vi "4Pi Focus Lock.vi"() -> ()   [LabVIEW 2016]
uses:
  4Pi Focus Lock Controls/4Pi Focus Lock - Notifier Type.ctl
  4Pi Focus Lock Controls/4Pi Focus Lock - Actions.ctl
  <vilib>/vision/Image Controls.llb/IMAQ Image.ctl
  Hardware Configuration/Hardware Configuration Controls/Device Type.ctl
  Hardware Configuration/Hardware Configuration Controls/Device Function.ctl
  Device Library/Cameras/Camera Controls/Generic Camera ROI.ctl
  Device Library/Cameras/Camera Controls/Generic Camera Actions.ctl
  Device Library/Stages/Stages Controls/Stage Actions.ctl
  <vilib>/addons/control/pid/pid.llb/PID (DBL).vi
  <vilib>/vision/NI_Vision_Development_Module.lvlib
  <vilib>/addons/control/pid/NI_PID_pid.lvlib
panel:
  in  "Z Drift Threshold (µm)":dbl=2.0
  in  "Z Move Limit (µm)":dbl=2.0
  out "Z Move":bool
  in  "Update Scale Factor":dbl=2.0
  out "dz (µm)":dbl format="%.2f"
  out "dt (s)":dbl format="%.3f"
  out "Measured Z (µm)":dbl=1.0 format="%.3g"
  out "Target Z (µm)":dbl=1.0 format="%.3g"
  out "Stage Position (µm)":dbl=1.0 format="%.2g"
  in  "Quit":bool
  in  "Sample Z Step No.":u32=2
  in  "Sample Z Step Size (µm)":dbl=2.0
  in  "D (Derivative)":dbl
  in  "I (Integral)":dbl
  in  "P (Proportional)":dbl=2.0
  in  "Set Camera ROI":bool
  out "Z Target and Fit Value (µm)":T1(graph)
  in  "Start Lock":bool
  # "PID Control Values"
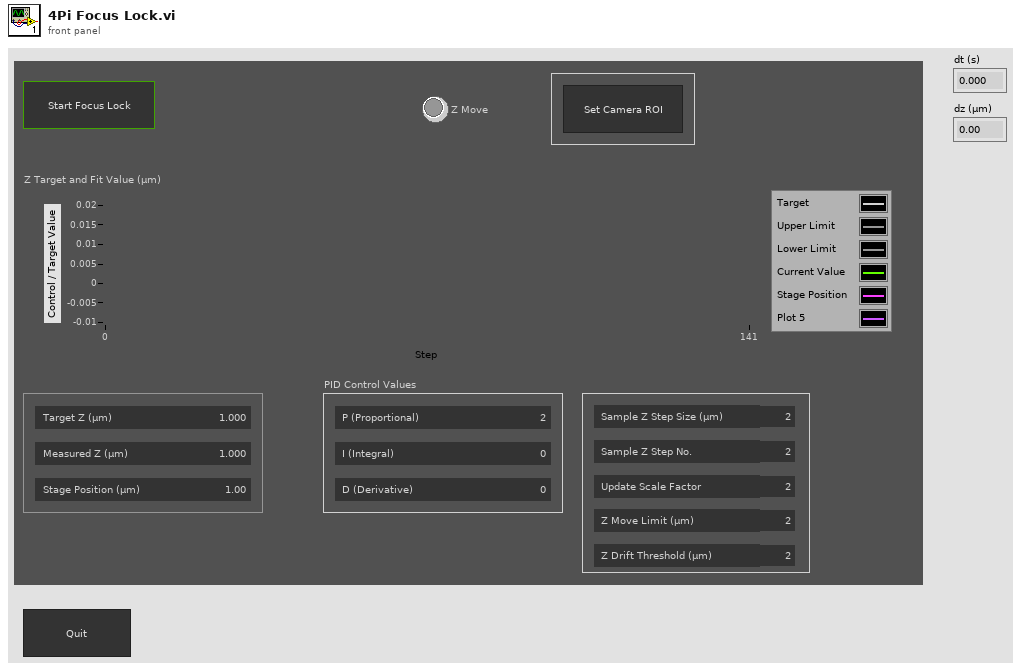
[diagram p1: front panel]
types:
  T1 = cluster{"Target 01":dbl, dbl, dbl, "Current 01":dbl, "Stage Position":dbl}
  T2 = typedef "4Pi Focus Lock - Actions.ctl" = enum16{"Idle", "Start Lock", "Restart Lock", "Get Target Position", "Get Ref Stack", "Cal Ref FFT", "Move To Init Z", "Start Primary Camera", "Get Current Position", "Get Current Position 1", "Get Actual Position", "Check Drift", "Move Z", "Update Plots", "Delay", "Abort", "Exit Loop", "Quit"}
  T3 = typedef "4Pi Focus Lock - Notifier Type.ctl" = cluster{"Actions":T2, "Z Drift Threshold":dbl, "Z Stage Move Limit (µm)":dbl, "Abort If Error":bool, "Z Correction Active":bool, "PID Values":dbl[], "Running?":bool, "Update Delay (ms)":i32, "Z Step Size (µm)":dbl, "Z Step No.":u32, "No. of Frames":u32, "Ref Stack (SGL)":T4[], "Cur Image (SGL)":T4, "Tmp Image FFT (CSG) ":T4, "Cur Image FFT (CSG) ":T4, "CC Image (SGL) ":T4, "Sample Z (µm)":dbl[], "Initial Z Position (µm)":dbl, "Ref FFT Stack (CSG)":T4[], "Tmp Image1 FFT (CSG) ":T4}
  T4 = typedef "IMAQ Image.ctl" = refnum<image>
  T5 = typedef "Image Type" = u32
  T6 = typedef "Device Function.ctl" = enum16{"Primary", "Secondary", "Overview", "Wide Field Drift Correction", "642 nm Excitation", "560 nm Excitation", "940 nm Excitation", "546 nm Excitation", "488 nm Excitation", "405 nm Excitation", "Objective Drift Correction", "4Pi Focus Lock", "4Pi Objective Lock", "Objective XY", "Objective Z", "Sample XY", "Sample Coarse Z", "Sample Z", "4Pi Lower", "4Pi Upper", "Mojo", "Adj Cavity", "Line Scanning", "Alert"}
  T7 = typedef "Device Type.ctl" = enum16{"AOTF", "Camera", "Deformable Mirror", "Laser", "Shutter", "Stage", "Waveform", "FPGA", "Email"}
  T8 = typedef "Stage Actions.ctl" = enum16{"Get Position", "MVR", "MOVE", "HALT", "ONTARGET", "ERROR", "REFERENCE", "INIT", "VELOCITY", "STATUS", "EXIT", "HOME", "ZEROPOS", "NANOPOS", "ANALOG", "QUIT"}
  T9 = typedef "Generic Camera Actions.ctl" = enum16{"Status", "Live Preview", "Capture", "Abort", "Set Exposure Time (s)", "Get Exposure Time (s)", "Record Settings", "Set ROI", "Get ROI", "Defect Correction On/Off", "Cooler On/Off", "Fan On/Off", "Quit"}
  T10 = typedef "Generic Camera ROI.ctl" = cluster{"H_Offset":u16, "V_Offset":u16, "H_Width":u16, "V_Width":u16}
  T11 = typedef "Stage Status.ctl" = enum16{"Error", "Abort", "Busy", "On Target"}
  T12 = cluster{"PID Values[0]":dbl, "PID Values[1]":dbl, "PID Values[2]":dbl}
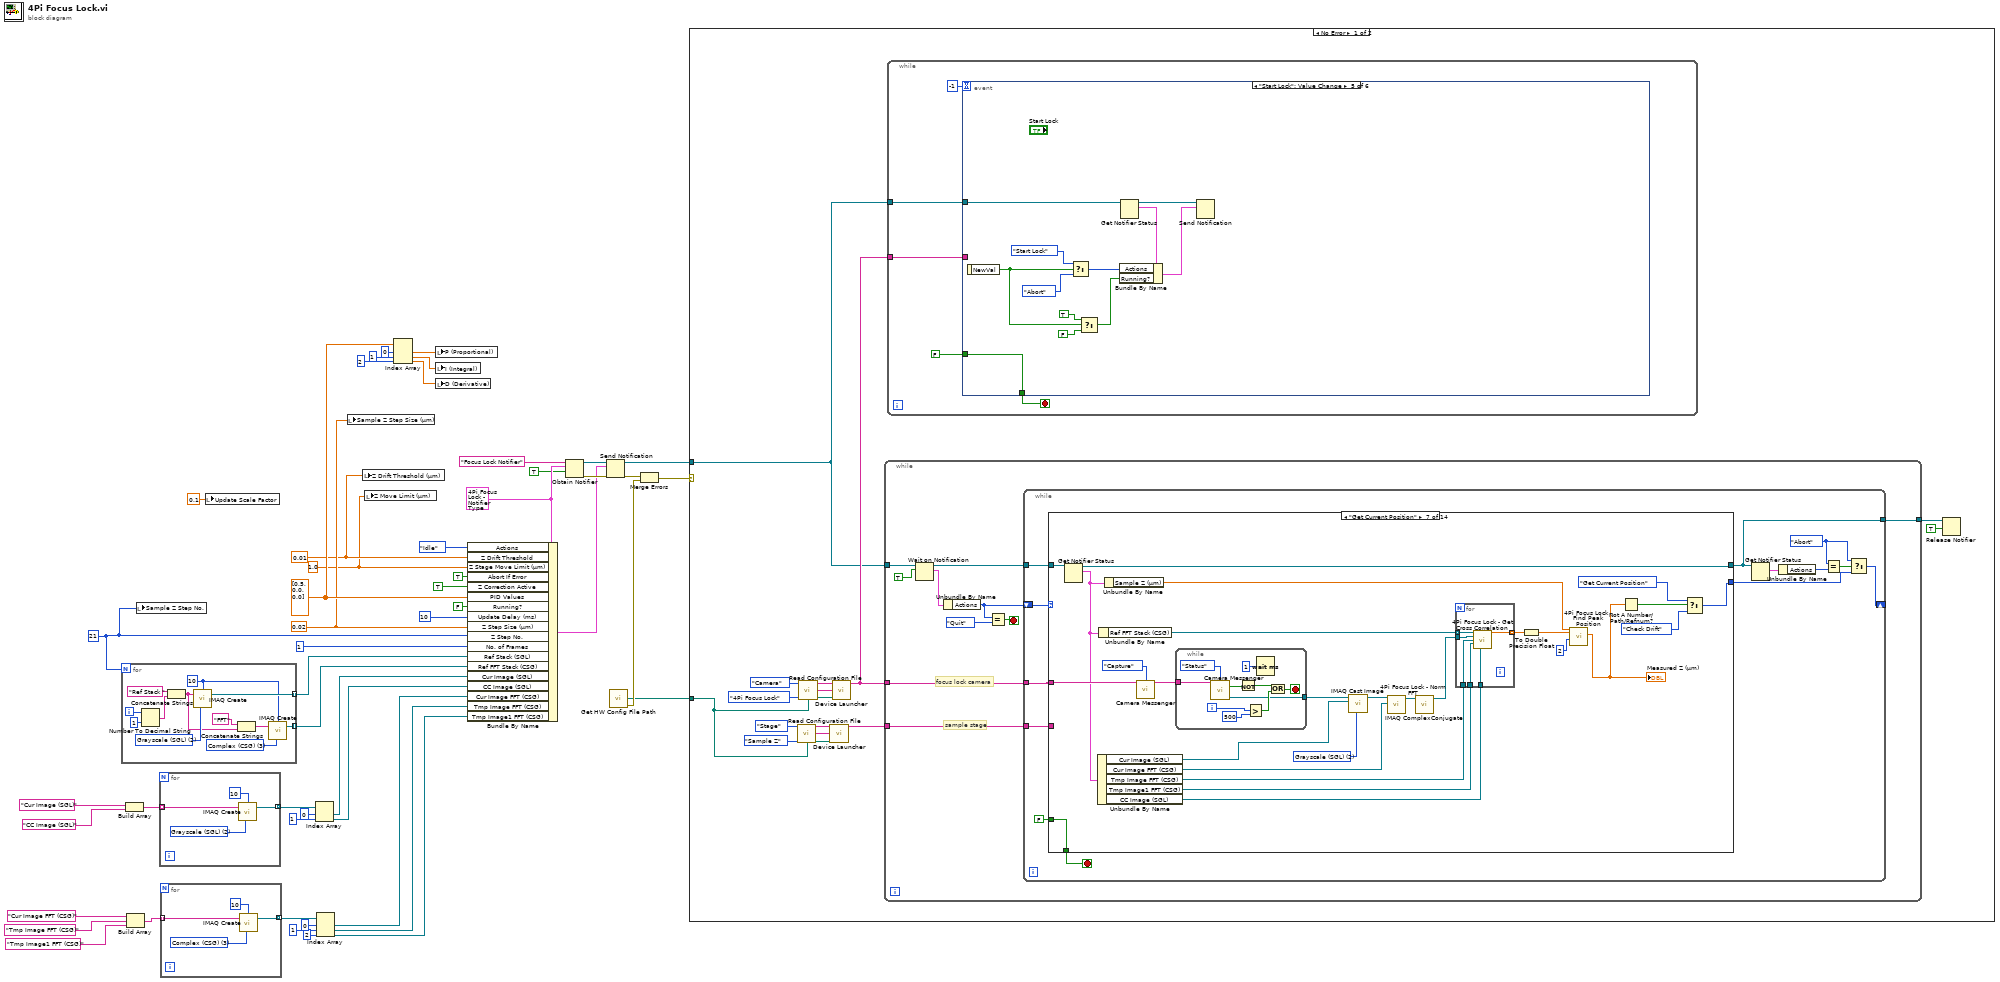
[diagram p0: block diagram]
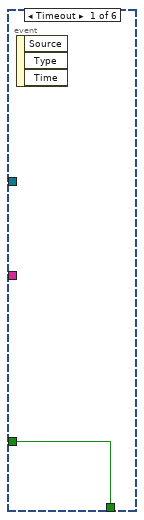
[diagram p2: hidden frame]
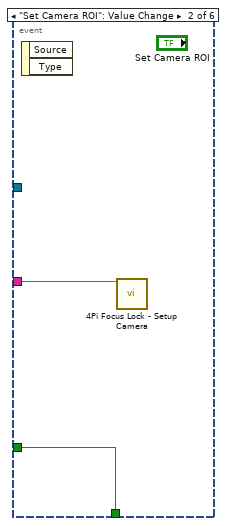
[diagram p3: hidden frame]
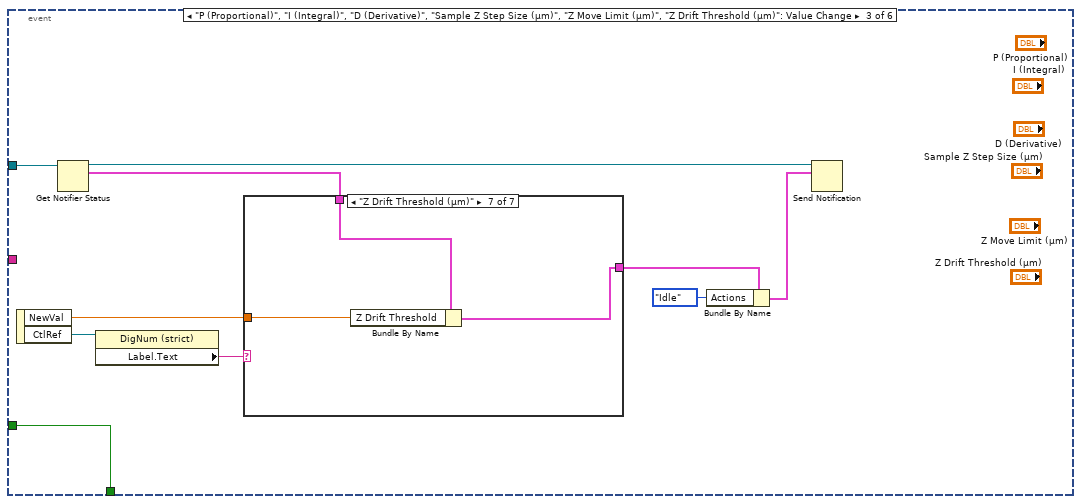
[diagram p4: hidden frame]
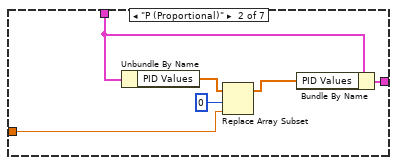
[diagram p6: hidden frame]
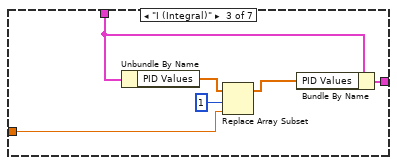
[diagram p7: hidden frame]
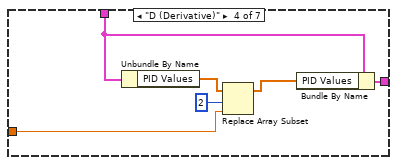
[diagram p8: hidden frame]
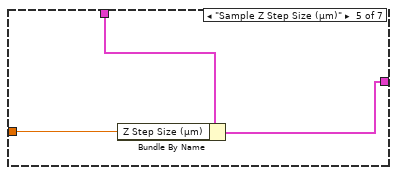
[diagram p9: hidden frame]
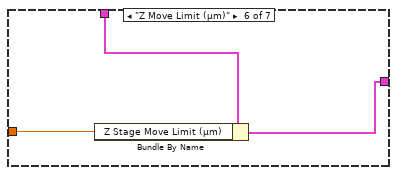
[diagram p10: hidden frame]
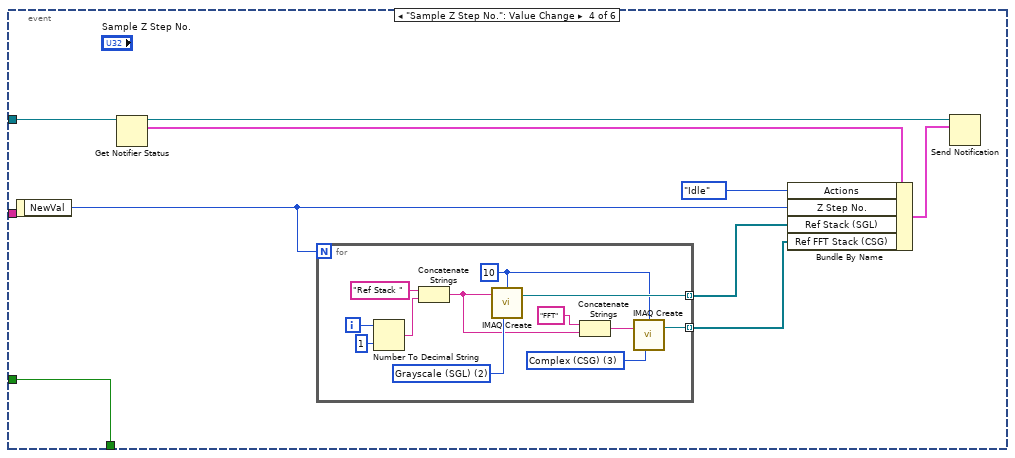
[diagram p11: hidden frame]
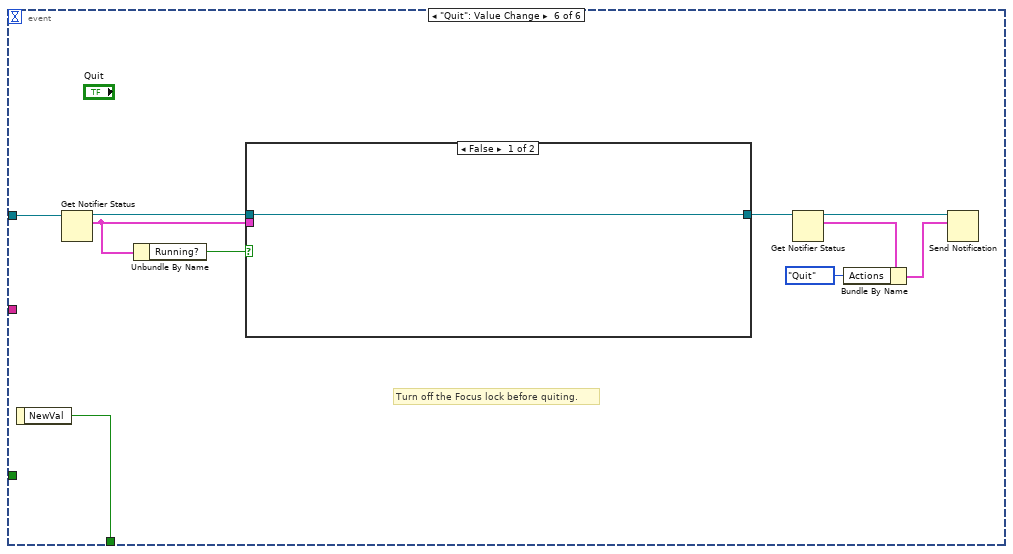
[diagram p12: hidden frame]
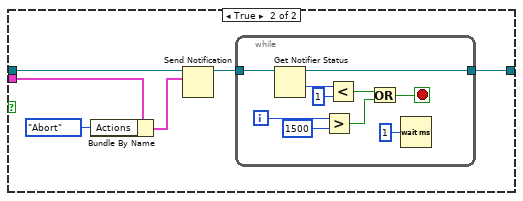
[diagram p13: hidden frame]
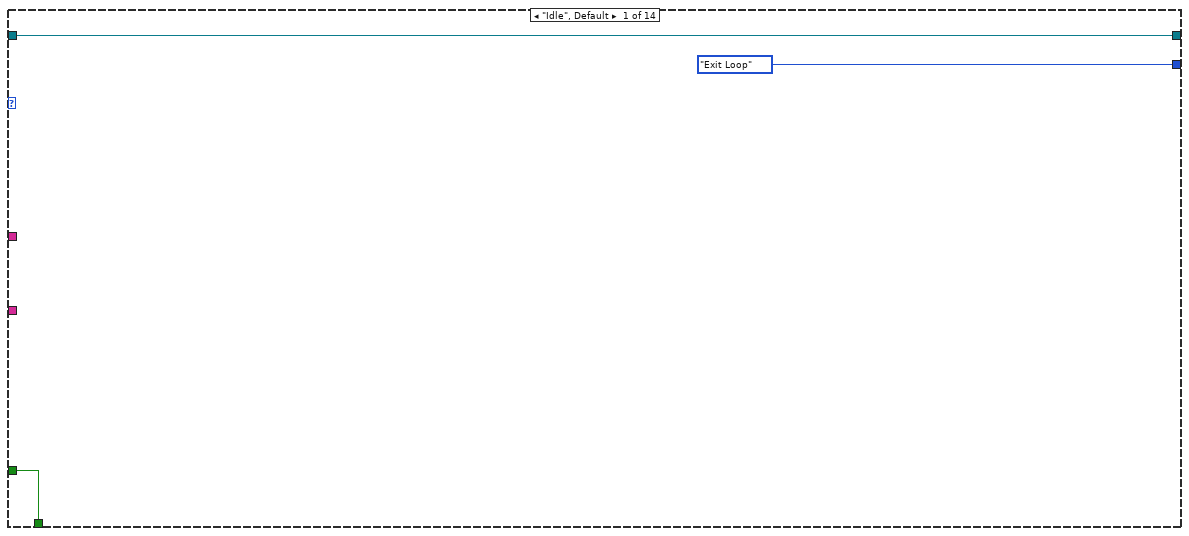
[diagram p14: hidden frame]
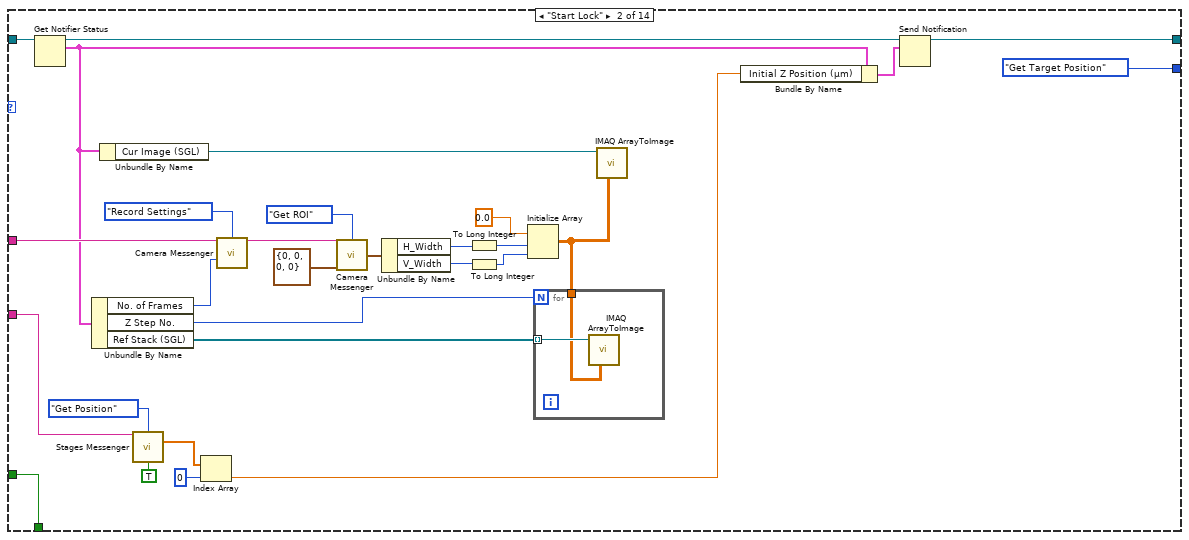
[diagram p15: hidden frame]
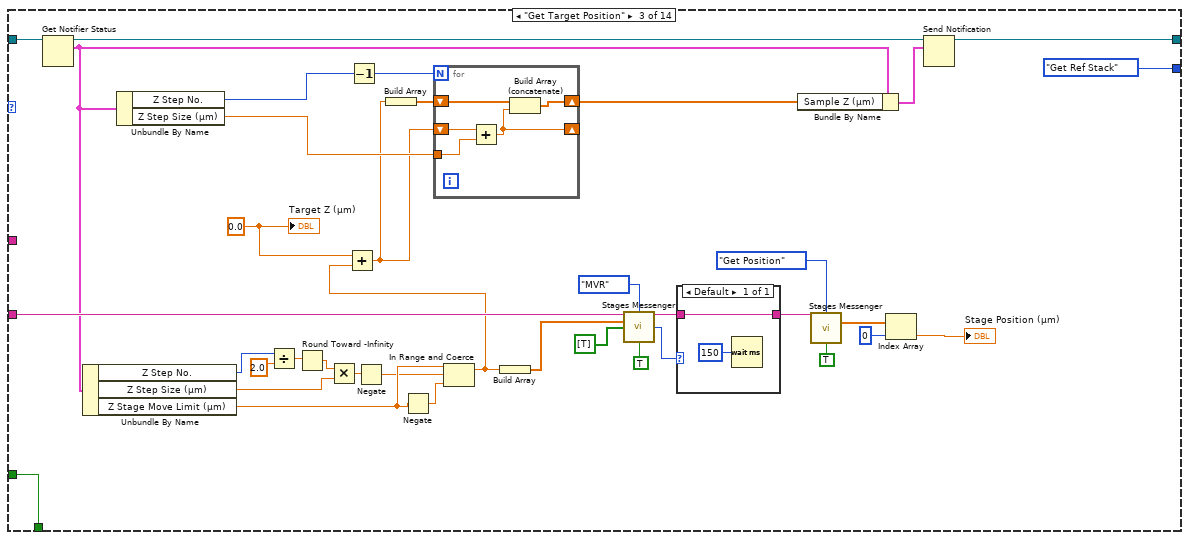
[diagram p16: hidden frame]
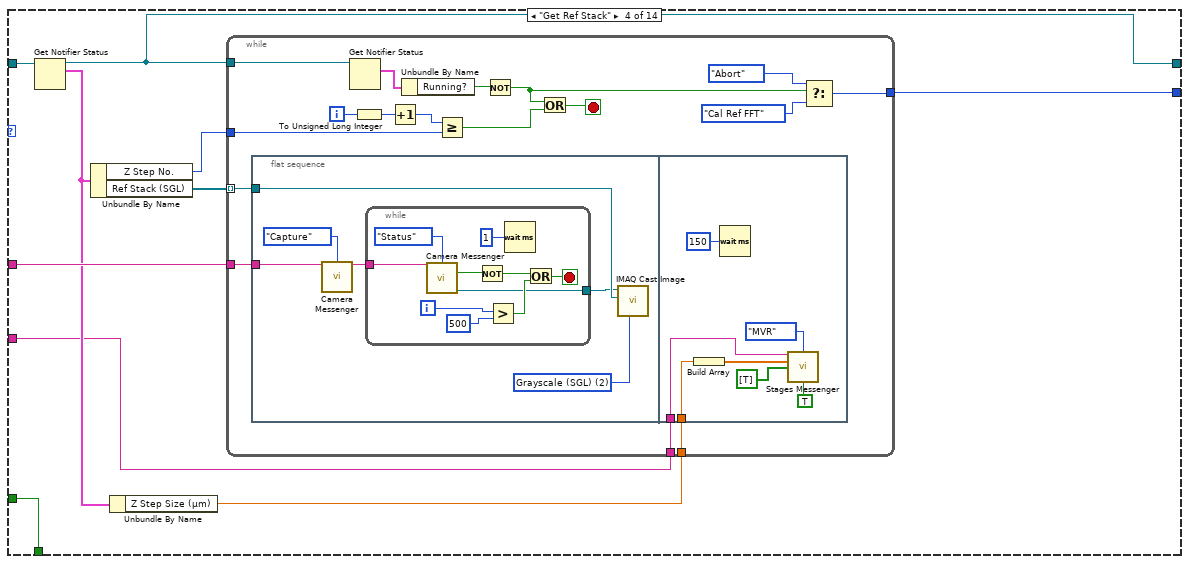
[diagram p17: hidden frame]
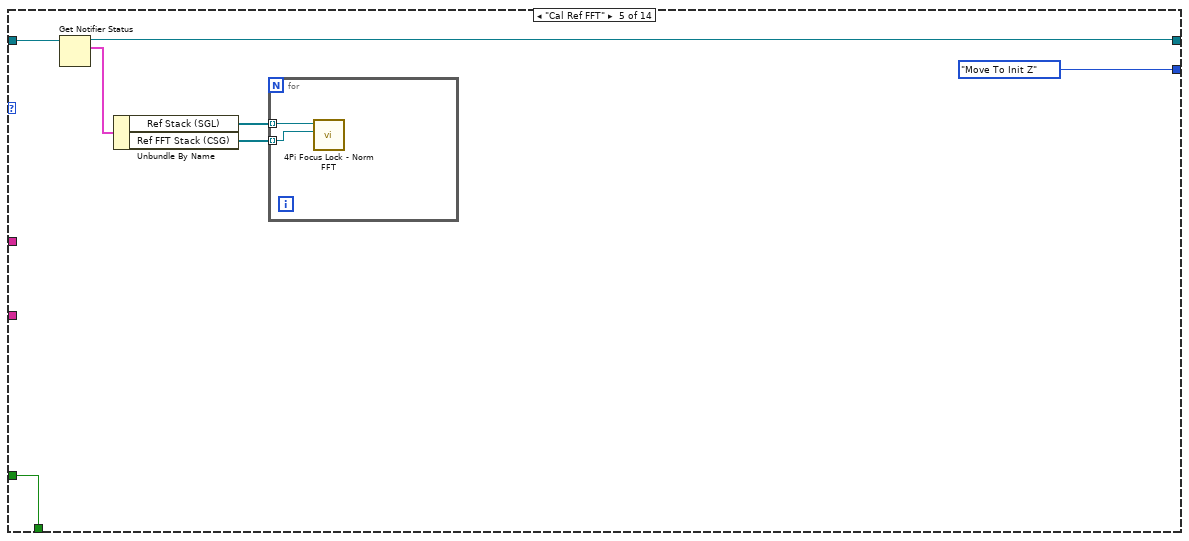
[diagram p18: hidden frame]
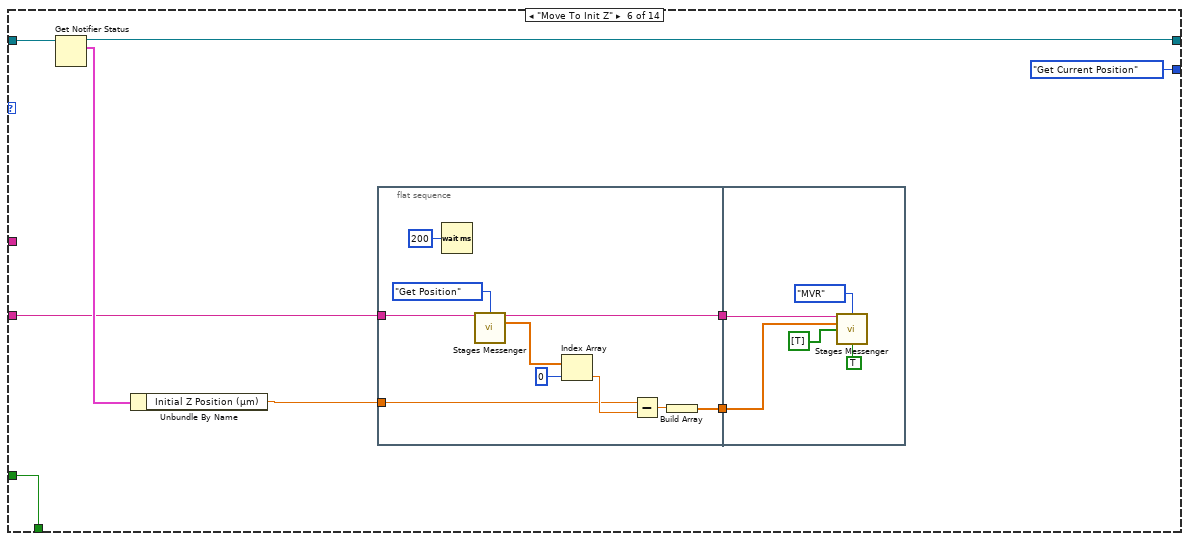
[diagram p19: hidden frame]
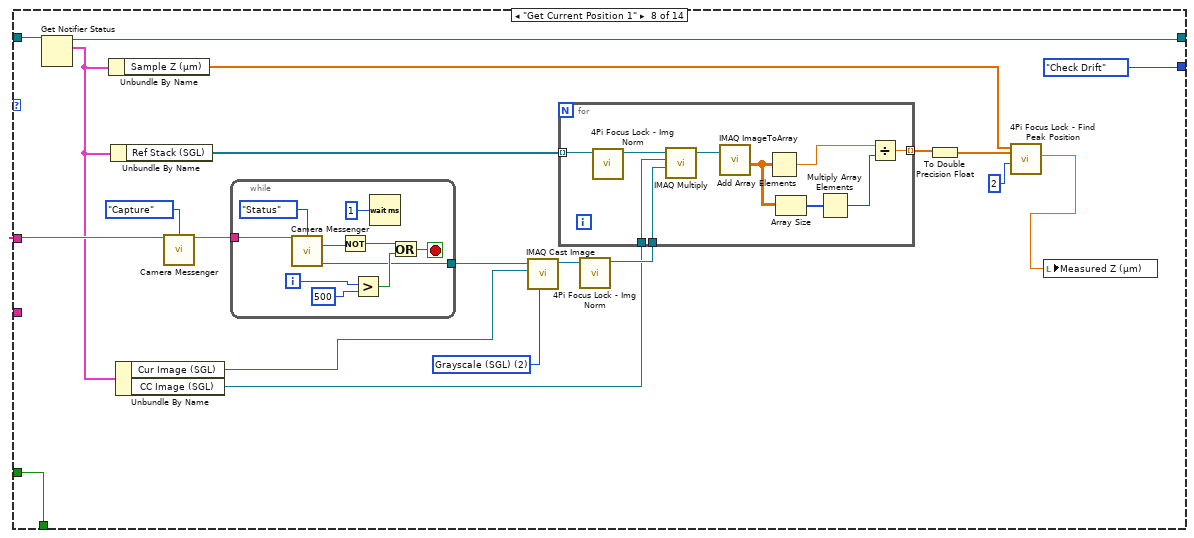
[diagram p20: hidden frame]
diagram:
  w28 = u32 21 ("Z Step No.")
  w35 = 0.02 ("Z Step Size (µm)")
  w39 = dbl[] [0.5, 0.0, 0.0] ("PID Values")
  w7 = 1.0 ("Z Stage Move Limit (µm)")
  w8 = 0.01 ("Z Drift Threshold")
  w10 = T3 {"Actions"=enum."Idle", "Z Drift Threshold"=0.05, "Z Stage Move Limit (µm)"=1.0, "Abort If Error"=FALSE, "Z Correction Active"=FALSE, "PID Values"=[], "Running?"=FALSE, "Update Delay (ms)"=0, "Z Step Size (µm)"=2.0, "Z Step No."=2, "No. of Frames"=0, "Ref Stack (SGL)"=[], "Cur Image (SGL)"=refnum, "Tmp Image FFT (CSG) "=refnum, "Cur Image FFT (CSG) "=refnum, "CC Image (SGL) "=refnum, "Sample Z (µm)"=[], "Initial Z Position (µm)"=0.0, "Ref FFT Stack (CSG)"=[], "Tmp Image1 FFT (CSG) "=refnum} ("4Pi Focus Lock")
  n1 = for {
    N: w28 -> [_]
    tunnel: [w62] -> w27 mode=indexing
    tunnel: [w51] -> w4 mode=indexing
    i -> [w61]
    w56 = T5 3 items=["Grayscale (U8)", "Grayscale (I16)", "Grayscale (SGL)", "Complex (CSG)", "RGB (U32)", "HSL (U32)", "RGB (U64)", "Grayscale (U16)"] ("Image Type")
    w57 = T5 2 items=["Grayscale (U8)", "Grayscale (I16)", "Grayscale (SGL)", "Complex (CSG)", "RGB (U32)", "HSL (U32)", "RGB (U64)", "Grayscale (U16)"] ("Image Type")
    w53 = 10 ("Border Size")
    n2 = Number To Decimal String(number=w61, width (-)=i16 1) -> (decimal integer string=w59:string)
    n3 = Concatenate Strings("Ref Stack " ("string"), w59) -> (w52:string)
    n4 = call "IMAQ Create"("Border Size"=w53, "Image Name"=w52, "Image Type"=w57) -> ("New Image"=w62:T4)  [unwired: 2 in, 1 out]
    n5 = Concatenate Strings("FFT" ("string"), w52) -> (w55:string)
    n6 = call "IMAQ Create"("Border Size"=w53, "Image Name"=w55, "Image Type"=w56) -> ("New Image"=w51:T4)  [unwired: 2 in, 1 out]
  }
  n7 = Build Array("Cur Image (SGL)" ("Image Name"), "CC Image (SGL)" ("Image Name")) -> (w22:string[])
  n8 = Build Array("Cur Image FFT (CSG)" ("Image Name"), "Tmp Image FFT (CSG)" ("Image Name"), "Tmp Image1 FFT (CSG)" ("Image Name")) -> (w14:string[])
  n9 = local write "Sample Z Step No."(w28) -> ()
  n10 = for {
    tunnel: w22 -> [w64] mode=indexing
    tunnel: [w63] -> w21 mode=indexing
    w65 = T5 2 items=["Grayscale (U8)", "Grayscale (I16)", "Grayscale (SGL)", "Complex (CSG)", "RGB (U32)", "HSL (U32)", "RGB (U64)", "Grayscale (U16)"] ("Image Type")
    n11 = call "IMAQ Create"("Border Size"=10, "Image Name"=w64, "Image Type"=w65) -> ("New Image"=w63:T4)  [unwired: 2 in, 1 out]
  }
  n12 = for {
    tunnel: w14 -> [w68] mode=indexing
    tunnel: [w67] -> w13 mode=indexing
    w69 = T5 3 items=["Grayscale (U8)", "Grayscale (I16)", "Grayscale (SGL)", "Complex (CSG)", "RGB (U32)", "HSL (U32)", "RGB (U64)", "Grayscale (U16)"] ("Image Type")
    n13 = call "IMAQ Create"("Border Size"=10, "Image Name"=w68, "Image Type"=w69) -> ("New Image"=w67:T4)  [unwired: 2 in, 1 out]
  }
  n14 = local write "Update Scale Factor"(0.1 ("Update Scale Factor")) -> ()
  n15 = Index Array(array=w21, index #1=0 ("index"), index #2=1 ("index")) -> (element #1=w20:T4, element #2=w19:T4)
  n16 = Index Array(array=w13, index #1=0 ("index"), index #2=1 ("index"), index #3=2 ("index")) -> (element #1=w12:T4, element #2=w11:T4, element #3=w1:T4)
  n17 = local write "Sample Z Step Size (µm)"(w35) -> ()
  n18 = local write "Z Drift Threshold (µm)"(w8) -> ()
  n19 = local write "Z Move Limit (µm)"(w7) -> ()
  n20 = Index Array(array=w39, index #1=0 ("index"), index #2=1 ("index"), index #3=2 ("index")) -> (element #1=w38:dbl, element #2=w37:dbl, element #3=w36:dbl)
  n21 = local write "P (Proportional)"(w38) -> ()
  n22 = local write "I (Integral)"(w37) -> ()
  n23 = local write "D (Derivative)"(w36) -> ()
  n24 = Bundle By Name(cluster=w10, "Actions"=4Pi_Focus_Lock_-_Actions."Idle", "Z Drift Threshold"=w8, "Z Stage Move Limit (µm)"=w7, "Abort If Error"=TRUE, "Z Correction Active"=TRUE, "PID Values"=w39, "Running?"=FALSE, "Update Delay (ms)"=10, "Z Step Size (µm)"=w35, "Z Step No."=w28, "No. of Frames"=u32 1, "Ref Stack (SGL)"=w27, "Ref FFT Stack (CSG)"=w4, "Cur Image (SGL)"=w20, "CC Image (SGL)"=w19, "Cur Image FFT (CSG)"=w12, "Tmp Image FFT (CSG)"=w11, "Tmp Image1 FFT (CSG)"=w1) -> (w5:T3)
  n25 = Obtain Notifier(name (unnamed)="Focus Lock Notifier", notification data type=w10, create if not found? (T)=TRUE) -> (notifier out=w44:refnum<notifier>, error out=w43:errorcluster)  [unwired: 1 in, 1 out]
  n26 = Send Notification(notification=w5, notifier=w44, error in (no error)=w43) -> (notifier out=w30:refnum<notifier>, error out=w34:errorcluster)
  n27 = call "Get HW Config File Path.vi"() -> ("File Path"=w32:path, "Error"=w33:errorcluster)  [unwired: 14 in]
  n28 = Merge Errors(w34, w33) -> (w31:errorcluster)
  n29 = case shown="No Error" w31 {
    tunnel: w32 -> [w71 _]
    tunnel: w30 -> [w74 _]
    frame No Error {
      n30 = call "Read Configuration File.vi"("Device Type"=Device_Type."Stage", "Device Function"=Device_Function."Sample Z", "Config File Path"=w71) -> ("Unique Notifier Name"=w81:string, "Device Ports/IDs/Channels"=w79:string[], "Device Engine Path"=w78:path)  [unwired: 9 in, 1 out]
      n31 = call "Read Configuration File.vi"("Device Type"=Device_Type."Camera", "Device Function"=Device_Function."4Pi Focus Lock", "Config File Path"=w71) -> ("Unique Notifier Name"=w86:string, "Device Ports/IDs/Channels"=w85:string[], "Device Engine Path"=w84:path)  [unwired: 9 in, 1 out]
      n32 = call "Device Launcher.vi"("Notifier Name"=w81, "Device Ports/IDs/Channels"=w79, "Device Engine Path"=w78) -> ("Notifier Name"=w76:string)  [unwired: 11 in, 1 out]
      n33 = call "Device Launcher.vi"("Notifier Name"=w86, "Device Ports/IDs/Channels"=w85, "Device Engine Path"=w84) -> ("Notifier Name"=w75:string)  [unwired: 11 in, 1 out]
      n34 = while {
        tunnel: w74 -> [w202]
        tunnel: w75 -> [w196]
        tunnel: w76 -> [w195]
        tunnel: [w193] -> w72
        stop <- w198 stop-if-true
        # "sample stage"
        # "focus lock camera"
        n35 = Wait on Notification(notifier=w202, ignore previous (F)=TRUE) -> (notifier out=w194:refnum<notifier>, notification=w200:T3)  [unwired: 2 in, 2 out]
        n36 = Unbundle By Name(w200) -> ("Actions"=w197:T2)
        n37 = Equal?(x=w197, y=4Pi_Focus_Lock_-_Actions."Quit") -> (x = y?=w198:bool)
        n38 = while {
          tunnel: w196 -> [w214]
          tunnel: w195 -> [w213]
          tunnel: w194 -> [w212]
          shift-right: [w206] -> _
          shift-left: w197 -> [w215]
          tunnel: [w203] -> w193
          stop <- w205 stop-if-true
          w208 = 4Pi_Focus_Lock_-_Actions."Abort" ("y")
          n39 = case shown="\"Get Current Position\"" w215 {
            tunnel: w214 -> [_ w238 _ w302 _ _ w402 w438 _ _ _ w520 _ _]
            tunnel: w213 -> [_ w227 w281 w294 _ w356 _ _ _ w484 w503 _ _ _]
            tunnel: w212 -> [w216 w240 w282 w303 w349 w361 w401 w437 w471 w489 w513 w521 w528 w532]
            tunnel: [4Pi_Focus_Lock_-_Actions."Exit Loop" ("y") 4Pi_Focus_Lock_-_Actions."Get Target Position" ("y") 4Pi_Focus_Lock_-_Actions."Get Ref Stack" ("y") w295 4Pi_Focus_Lock_-_Actions."Move To Init Z" ("y") 4Pi_Focus_Lock_-_Actions."Get Current Position" ("y") w377 4Pi_Focus_Lock_-_Actions."Check Drift" ("y") 4Pi_Focus_Lock_-_Actions."Move Z" ("y") w474 4Pi_Focus_Lock_-_Actions."Get Current Position" ("y") 4Pi_Focus_Lock_-_Actions."Exit Loop" ("y") 4Pi_Focus_Lock_-_Actions."Exit Loop" ("y") 4Pi_Focus_Lock_-_Actions."Quit" ("y")] -> w207
            tunnel: [w216 w221 w269 w297 w346 w359 w393 w431 w461 w482 w501 w517 w528 w532] -> w203
            tunnel: [w217 w220 w268 w296 w344 w357 w392 w430 w460 w481 w500 w516 TRUE TRUE] -> w205
            tunnel: FALSE -> [w217 w220 w268 w296 w344 w357 w392 w430 w460 w481 w500 w516 _ _]
            frame "Idle", Default {
            }
            frame "Start Lock" {
              n40 = Get Notifier Status(notifier=w240) -> (notifier out=w223:refnum<notifier>, current notification=w226:T3)  [unwired: 1 in, 3 out]
              n41 = Unbundle By Name(w226) -> ("No. of Frames"=w235:u32, "Z Step No."=w234:u32, "Ref Stack (SGL)"=w233:T4[])
              n42 = Unbundle By Name(w226) -> ("Cur Image (SGL)"=w231:T4)
              n43 = call "Stages Messenger.vi"("Stage Notifier Name"=w227, "Actions"=Stage_Actions."Get Position", "Exit While Busy?"=TRUE) -> ("Positions"=w228:dbl[])  [unwired: 9 in, 3 out]
              n44 = Index Array(array=w228, index=0) -> (element=w225:dbl)
              n45 = call "Camera Messenger.vi"("Notifier Name"=w238, "General Camera Actions"=Generic_Camera_Actions."Record Settings", "No. of Frames"=w235) -> ("Notifier Name Dup"=w236:string)  [unwired: 7 in, 5 out]
              n46 = call "Camera Messenger.vi"("Notifier Name"=w236, "General Camera Actions"=Generic_Camera_Actions."Get ROI", "Camera ROI"=T10 {"H_Offset"=0, "V_Offset"=0, "H_Width"=0, "V_Width"=0} ("General Camera ROI")) -> ("Camera ROI"=w245:T10)  [unwired: 7 in, 5 out]
              n47 = Unbundle By Name(w245) -> ("H_Width"=w244:u16, "V_Width"=w242:u16)
              n48 = To Long Integer(number=w244) -> (32bit integer=w243:i32)
              n49 = To Long Integer(number=w242) -> (32bit integer=w241:i32)
              n50 = Initialize Array(sgl 0.0 ("element"), w243, w241) -> (w232:sgl[][])
              n51 = for {
                N: w234 -> [_]
                tunnel: w232 -> [w248]
                tunnel: w233 -> [w249] mode=indexing
                n52 = call "IMAQ ArrayToImage"("Image Pixels (Float)"=w248, "Image"=w249) -> ()  [unwired: 8 in, 2 out]
              }
              n53 = call "IMAQ ArrayToImage"("Image Pixels (Float)"=w232, "Image"=w231) -> ()  [unwired: 8 in, 2 out]
              n54 = Bundle By Name(cluster=w226, "Initial Z Position (µm)"=w225) -> (w224:T3)
              n55 = Send Notification(notification=w224, notifier=w223) -> (notifier out=w221:refnum<notifier>)  [unwired: 1 in, 1 out]
            }
            frame "Get Target Position" {
              w275 = 0.0 ("Target Z (µm)")
              n56 = Get Notifier Status(notifier=w282) -> (notifier out=w273:refnum<notifier>, current notification=w278:T3)  [unwired: 1 in, 3 out]
              n57 = Unbundle By Name(w278) -> ("Z Step No."=w267:u32, "Z Step Size (µm)"=w266:dbl, "Z Stage Move Limit (µm)"=w264:dbl)
              n58 = Unbundle By Name(w278) -> ("Z Step No."=w259:u32, "Z Step Size (µm)"=w276:dbl)
              n59 = Divide(x=w267, y=2.0) -> (x/y=w257:dbl)
              n60 = Round Toward -Infinity(1:w257) -> (0:w256:dbl)
              n61 = Multiply(x=w256, y=w266) -> (x*y=w261:dbl)
              n62 = Decrement(x=w259) -> (x-1=w258:u32)
              n63 = Negate(x=w261) -> (-x=w260:dbl)
              n64 = Negate(x=w264) -> (-x=w265:dbl)
              n65 = In Range and Coerce(upper limit=w264, x=w260, lower limit=w265) -> (coerced(x)=w262:dbl)  [unwired: 1 out]
              n66 = Add(x=w275, y=w262) -> (x+y=w263:dbl)
              n67 = Build Array(w263) -> (w277:dbl[])
              n68 = for {
                N: w258 -> [_]
                tunnel: w276 -> [w291]
                shift-right: [w292] -> w274
                shift-left: w277 -> [w293]
                shift-right: [w289] -> _
                shift-left: w263 -> [w290]
                n69 = Add(x=w290, y=w291) -> (x+y=w289:dbl)
                n70 = Build Array (concatenate)(w293, w289) -> (w292:dbl[])
              }
              n71 = Build Array(w262) -> (w279:dbl[])
              n72 = call "Stages Messenger.vi"("Stage Notifier Name"=w281, "Actions"=Stage_Actions."MVR", "Setpoint"=w279, "Axis"=bool[] [TRUE], "Exit While Busy?"=TRUE) -> ("Stage Notifier Name (Dup)"=w254:string, "Status"=w255:T11)  [unwired: 7 in, 2 out]
              n73 = case shown="Default" w255 {
                tunnel: [w287] -> w253
                tunnel: w254 -> [w287]
                frame Default {
                  n74 = Wait (ms)(milliseconds to wait=u32 150) -> ()  [unwired: 1 out]
                }
              }
              n75 = Bundle By Name(cluster=w278, "Sample Z (µm)"=w274) -> (w272:T3)
              n76 = call "Stages Messenger.vi"("Stage Notifier Name"=w253, "Actions"=Stage_Actions."Get Position", "Exit While Busy?"=TRUE) -> ("Positions"=w251:dbl[])  [unwired: 9 in, 3 out]
              n77 = Index Array(array=w251, index=0) -> (element=→"Stage Position (µm)":dbl)
              n78 = Send Notification(notification=w272, notifier=w273) -> (notifier out=w269:refnum<notifier>)  [unwired: 1 in, 1 out]
              "Target Z (µm)" <- w275
            }
            frame "Get Ref Stack" {
              n79 = Get Notifier Status(notifier=w303) -> (notifier out=w297:refnum<notifier>, current notification=w301:T3)  [unwired: 1 in, 3 out]
              n80 = Unbundle By Name(w301) -> ("Z Step No."=w300:u32, "Ref Stack (SGL)"=w299:T4[])
              n81 = Unbundle By Name(w301) -> ("Z Step Size (µm)"=w298:dbl)
              n82 = while {
                tunnel: w302 -> [w320]
                tunnel: w300 -> [w317]
                tunnel: w297 -> [w319]
                tunnel: [w307] -> w295
                tunnel: w299 -> [w306] mode=indexing
                tunnel: w298 -> [w305]
                tunnel: w294 -> [w304]
                i -> [w316]
                stop <- w312 stop-if-true
                n83 = flat-sequence {
                  tunnel: w320 -> [w326]
                  tunnel: w306 -> [w323]
                  tunnel: w305 -> [w338]
                  tunnel: w304 -> [w337]
                  frame #0 {
                    w324 = T5 2 items=["Grayscale (U8)", "Grayscale (I16)", "Grayscale (SGL)", "Complex (CSG)", "RGB (U32)", "HSL (U32)", "RGB (U64)", "Grayscale (U16)"] ("Image Type")
                    n84 = call "Camera Messenger.vi"("Notifier Name"=w326, "General Camera Actions"=Generic_Camera_Actions."Capture") -> ("Notifier Name Dup"=w322:string)  [unwired: 8 in, 5 out]
                    n85 = while {
                      tunnel: w322 -> [w336]
                      tunnel: [w329] -> w321
                      i -> [w332]
                      stop <- w330 stop-if-true
                      n86 = call "Camera Messenger.vi"("Notifier Name"=w336, "General Camera Actions"=Generic_Camera_Actions."Status") -> ("Running?"=w328:bool, "Image Ref"=w329:T4)  [unwired: 8 in, 4 out]
                      n87 = Not(x=w328) -> (.not. x?=w327:bool)
                      n88 = Greater?(x=w332, y=500) -> (0:w334:bool)
                      n89 = Wait (ms)(milliseconds to wait=u32 1) -> ()  [unwired: 1 out]
                      n90 = Or(x=w327, y=w334) -> (x .or. y?=w330:bool)
                    }
                    n91 = call "IMAQ Cast Image"("Image Type"=w324, "Image Dst"=w323, "Image Src"=w321) -> ()  [unwired: 7 in, 2 out]
                  }
                  frame #1 {
                    n92 = Build Array(w338) -> (w342:dbl[])
                    n93 = Wait (ms)(milliseconds to wait=u32 150) -> ()  [unwired: 1 out]
                    n94 = call "Stages Messenger.vi"("Stage Notifier Name"=w337, "Actions"=Stage_Actions."MVR", "Setpoint"=w342, "Axis"=bool[] [TRUE], "Exit While Busy?"=TRUE) -> ()  [unwired: 7 in, 4 out]
                  }
                }
                n95 = Get Notifier Status(notifier=w319) -> (current notification=w311:T3)  [unwired: 1 in, 4 out]
                n96 = To Unsigned Long Integer(number=w316) -> (unsigned 32bit integer=w315:u32)
                n97 = Increment(x=w315) -> (x+1=w318:u32)
                n98 = Unbundle By Name(w311) -> ("Running?"=w314:bool)
                n99 = Greater Or Equal?(x=w318, y=w317) -> (x >= y?=w313:bool)
                n100 = Not(x=w314) -> (.not. x?=w310:bool)
                n101 = Or(x=w310, y=w313) -> (x .or. y?=w312:bool)
                n102 = Select(t=4Pi_Focus_Lock_-_Actions."Abort", s=w310, f=4Pi_Focus_Lock_-_Actions."Cal Ref FFT" ("y")) -> (s? t:f=w307:T2)
              }
            }
            frame "Cal Ref FFT" {
              n103 = Get Notifier Status(notifier=w349) -> (notifier out=w346:refnum<notifier>, current notification=w350:T3)  [unwired: 1 in, 3 out]
              n104 = Unbundle By Name(w350) -> ("Ref Stack (SGL)"=w347:T4[], "Ref FFT Stack (CSG)"=w348:T4[])
              n105 = for {
                tunnel: w348 -> [w351] mode=indexing
                tunnel: w347 -> [w352] mode=indexing
                n106 = call "4Pi Focus Lock - Norm FFT.vi"("FFT Image Dst"=w351, "Image In"=w352) -> ()  [unwired: 8 in, 2 out]
              }
            }
            frame "Move To Init Z" {
              n107 = Get Notifier Status(notifier=w361) -> (notifier out=w359:refnum<notifier>, current notification=w360:T3)  [unwired: 1 in, 3 out]
              n108 = Unbundle By Name(w360) -> ("Initial Z Position (µm)"=w354:dbl)
              n109 = flat-sequence {
                tunnel: w356 -> [w369]
                tunnel: [w368] -> w355
                tunnel: w354 -> [w364]
                tunnel: [w362] -> w353
                tunnel: w355 -> [w373]
                tunnel: w353 -> [w372]
                frame #0 {
                  n110 = Wait (ms)(milliseconds to wait=u32 200) -> ()  [unwired: 1 out]
                  n111 = call "Stages Messenger.vi"("Stage Notifier Name"=w369, "Actions"=Stage_Actions."Get Position") -> ("Stage Notifier Name (Dup)"=w368:string, "Positions"=w366:dbl[])  [unwired: 10 in, 2 out]
                  n112 = Index Array(array=w366, index=0) -> (element=w365:dbl)
                  n113 = Subtract(x=w364, y=w365) -> (x-y=w363:dbl)
                  n114 = Build Array(w363) -> (w362:dbl[])
                }
                frame #1 {
                  n115 = call "Stages Messenger.vi"("Stage Notifier Name"=w373, "Actions"=Stage_Actions."MVR", "Setpoint"=w372, "Axis"=bool[] [TRUE], "Exit While Busy?"=TRUE) -> ()  [unwired: 7 in, 4 out]
                }
              }
            }
            frame "Get Current Position" {
              w400 = T5 2 items=["Grayscale (U8)", "Grayscale (I16)", "Grayscale (SGL)", "Complex (CSG)", "RGB (U32)", "HSL (U32)", "RGB (U64)", "Grayscale (U16)"] ("Image Type")
              n116 = Get Notifier Status(notifier=w401) -> (notifier out=w393:refnum<notifier>, current notification=w397:T3)  [unwired: 1 in, 3 out]
              n117 = Unbundle By Name(w397) -> ("Cur Image (SGL)"=w389:T4, "Cur Image FFT (CSG)"=w384:T4, "Tmp Image FFT (CSG)"=w382:T4, "Tmp Image1 FFT (CSG)"=w383:T4, "CC Image (SGL)"=w398:T4)
              n118 = Unbundle By Name(w397) -> ("Ref FFT Stack (CSG)"=w388:T4[])
              n119 = Unbundle By Name(w397) -> ("Sample Z (µm)"=w395:dbl[])
              n120 = call "Camera Messenger.vi"("Notifier Name"=w402, "General Camera Actions"=Generic_Camera_Actions."Capture") -> ("Notifier Name Dup"=w391:string)  [unwired: 8 in, 5 out]
              n121 = while {
                tunnel: w391 -> [w419]
                tunnel: [w413] -> w390
                i -> [w415]
                stop <- w414 stop-if-true
                n122 = call "Camera Messenger.vi"("Notifier Name"=w419, "General Camera Actions"=Generic_Camera_Actions."Status") -> ("Running?"=w411:bool, "Image Ref"=w413:T4)  [unwired: 8 in, 4 out]
                n123 = Not(x=w411) -> (.not. x?=w410:bool)
                n124 = Greater?(x=w415, y=500) -> (0:w417:bool)
                n125 = Wait (ms)(milliseconds to wait=u32 1) -> ()  [unwired: 1 out]
                n126 = Or(x=w410, y=w417) -> (x .or. y?=w414:bool)
              }
              n127 = call "IMAQ Cast Image"("Image Type"=w400, "Image Dst"=w389, "Image Src"=w390) -> ("Image Dst Out"=w399:T4)  [unwired: 7 in, 1 out]
              n128 = call "4Pi Focus Lock - Norm FFT.vi"("FFT Image Dst"=w384, "Image In"=w399) -> ("FFT Image Out"=w386:T4)  [unwired: 8 in, 1 out]
              n129 = call "IMAQ ComplexConjugate"("Image Src"=w386) -> ("Image Dst Out"=w385:T4)  [unwired: 3 in, 1 out]
              n130 = for {
                tunnel: w398 -> [w409]
                tunnel: [w408] -> w396 mode=indexing
                tunnel: w385 -> [w407]
                tunnel: w388 -> [w406] mode=indexing
                tunnel: w383 -> [w405]
                tunnel: w382 -> [w404]
                n131 = call "4Pi Focus Lock - Get Cross Correlation.vi"("Ref FFT image"=w406, "Cur FFT Image"=w407, "FFT CC image"=w404, "iFFT image"=w405, "CC image"=w409) -> ("Max CC"=w408:sgl)  [unwired: 9 in, 1 out]
              }
              n132 = To Double Precision Float(number=w396) -> (double precision float=w387:dbl[])
              n133 = call "4Pi Focus Lock - Find Peak Position.vi"("Fit Size"=2, "y"=w387, "x"=w395) -> ("Coerced Peak Position"=w381:dbl)  [unwired: 7 in, 1 out]
              "Measured Z (µm)" <- w381
              n134 = Not A Number/Path/Refnum?(number/path/refnum=w381) -> (NaN/Path/Refnum?=w380:bool)
              n135 = Select(t=4Pi_Focus_Lock_-_Actions."Get Current Position", s=w380, f=4Pi_Focus_Lock_-_Actions."Check Drift" ("y")) -> (s? t:f=w377:T2)
            }
            frame "Get Current Position 1" {
              w436 = T5 2 items=["Grayscale (U8)", "Grayscale (I16)", "Grayscale (SGL)", "Complex (CSG)", "RGB (U32)", "HSL (U32)", "RGB (U64)", "Grayscale (U16)"] ("Image Type")
              n136 = Get Notifier Status(notifier=w437) -> (notifier out=w431:refnum<notifier>, current notification=w435:T3)  [unwired: 1 in, 3 out]
              n137 = Unbundle By Name(w435) -> ("Sample Z (µm)"=w434:dbl[])
              n138 = Unbundle By Name(w435) -> ("Ref Stack (SGL)"=w426:T4[])
              n139 = Unbundle By Name(w435) -> ("Cur Image (SGL)"=w427:T4, "CC Image (SGL)"=w422:T4)
              n140 = call "Camera Messenger.vi"("Notifier Name"=w438, "General Camera Actions"=Generic_Camera_Actions."Capture") -> ("Notifier Name Dup"=w429:string)  [unwired: 8 in, 5 out]
              n141 = while {
                tunnel: w429 -> [w459]
                tunnel: [w453] -> w428
                i -> [w455]
                stop <- w454 stop-if-true
                n142 = call "Camera Messenger.vi"("Notifier Name"=w459, "General Camera Actions"=Generic_Camera_Actions."Status") -> ("Running?"=w451:bool, "Image Ref"=w453:T4)  [unwired: 8 in, 4 out]
                n143 = Not(x=w451) -> (.not. x?=w450:bool)
                n144 = Greater?(x=w455, y=500) -> (0:w457:bool)
                n145 = Wait (ms)(milliseconds to wait=u32 1) -> ()  [unwired: 1 out]
                n146 = Or(x=w450, y=w457) -> (x .or. y?=w454:bool)
              }
              n147 = call "IMAQ Cast Image"("Image Type"=w436, "Image Dst"=w427, "Image Src"=w428) -> ("Image Dst Out"=w424:T4)  [unwired: 7 in, 1 out]
              n148 = call "4Pi Focus Lock - Img Norm.vi"("Image In"=w424) -> ("Image Dst Out"=w423:T4)  [unwired: 9 in, 1 out]
              n149 = for {
                tunnel: w426 -> [w449] mode=indexing
                tunnel: w423 -> [w447]
                tunnel: w422 -> [w446]
                tunnel: [w445] -> w421 mode=indexing
                n150 = call "4Pi Focus Lock - Img Norm.vi"("Image In"=w449) -> ("Image Dst Out"=w448:T4)  [unwired: 9 in, 1 out]
                n151 = call "IMAQ Multiply"("Image Src A"=w448, "Image Dst"=w446, "Image Src B"=w447) -> ("Image Dst Out"=w444:T4)  [unwired: 4 in, 1 out]
                n152 = call "IMAQ ImageToArray"("Image"=w444) -> ("Image Pixels (Float)"=w443:sgl[][])  [unwired: 3 in, 4 out]
                n153 = Add Array Elements(numeric array=w443) -> (sum=w441:sgl)
                n154 = Array Size(array=w443) -> (size(s)=w442:i32[])
                n155 = Multiply Array Elements(1:w442) -> (0:w440:i32)
                n156 = Divide(x=w441, y=w440) -> (x/y=w445:sgl)
              }
              n157 = To Double Precision Float(number=w421) -> (double precision float=w425:dbl[])
              n158 = call "4Pi Focus Lock - Find Peak Position.vi"("Fit Size"=2, "y"=w425, "x"=w434) -> ("Coerced Peak Position"=w420:dbl)  [unwired: 7 in, 1 out]
              n159 = local write "Measured Z (µm)"(w420) -> ()
            }
            frame "Check Drift" {
              n160 = Get Notifier Status(notifier=w471) -> (notifier out=w461:refnum<notifier>, current notification=w470:T3)  [unwired: 1 in, 3 out]
              n161 = local read "Measured Z (µm)"() -> (w472:dbl)
              n162 = Unbundle By Name(w470) -> ("Z Drift Threshold"=w464:dbl, "PID Values"=w469:dbl[])
              n163 = local read "Target Z (µm)"() -> (w473:dbl)
              n164 = Array To Cluster(array=w469) -> (cluster=w468:T12)
              n165 = call-poly <vilib>:"PID.vi"("PID gains"=w468, "process variable"=w472, "setpoint"=w473) -> ("dt out (s)"=→"dt (s)":dbl, "output"=w466:dbl)  [unwired: 7 in]
              "dz (µm)" <- w466
              n166 = Absolute Value(x=w466) -> (abs(x)=w465:dbl)
              n167 = Greater?(x=w465, y=w464) -> (0:→"Z Move":bool)
            }
            frame "Move Z" {
              n168 = Get Notifier Status(notifier=w489) -> (notifier out=w482:refnum<notifier>, current notification=w488:T3)  [unwired: 1 in, 3 out]
              n169 = Unbundle By Name(w488) -> ("Z Stage Move Limit (µm)"=w486:dbl)
              n170 = local read "dz (µm)"() -> (w487:dbl)
              n171 = Multiply(x=w487, y="Update Scale Factor") -> (x*y=w480:dbl)
              n172 = Absolute Value(x=w480) -> (abs(x)=w485:dbl)
              n173 = Greater?(x=w486, y=w485) -> (0:w476:bool)
              n174 = local read "Z Move"() -> (w478:bool)
              n175 = And(x=w476, y=w478) -> (x .and. y?=w479:bool)
              n176 = case shown="True" w479 {
                tunnel: w480 -> [_ w493]
                tunnel: w484 -> [_ w492]
                frame False {
                }
                frame True {
                  n177 = Build Array(w493) -> (w497:dbl[])
                  n178 = call "Stages Messenger.vi"("Stage Notifier Name"=w492, "Actions"=Stage_Actions."MVR", "Setpoint"=w497, "Axis"=bool[] [TRUE], "Exit While Busy?"=TRUE) -> ("Positions"=w495:dbl[])  [unwired: 7 in, 3 out]
                  n179 = Wait (ms)(milliseconds to wait=u32 50) -> ()  [unwired: 1 out]
                  n180 = Index Array(array=w495, index=0) -> ()  [unwired: 1 out]
                }
              }
              n181 = Select(t=4Pi_Focus_Lock_-_Actions."Update Plots" ("y"), s=w476, f=4Pi_Focus_Lock_-_Actions."Abort") -> (s? t:f=w474:T2)
            }
            frame "Update Plots" {
              n182 = Get Notifier Status(notifier=w513) -> (notifier out=w501:refnum<notifier>, current notification=w511:T3)  [unwired: 1 in, 3 out]
              n183 = Unbundle By Name(w511) -> ("Z Drift Threshold"=w512:dbl)
              n184 = Unbundle By Name(w511) -> ("Initial Z Position (µm)"=w510:dbl)
              n185 = call "Stages Messenger.vi"("Stage Notifier Name"=w503, "Actions"=Stage_Actions."Get Position", "Exit While Busy?"=TRUE) -> ("Positions"=w504:dbl[])  [unwired: 9 in, 3 out]
              n186 = local read "Measured Z (µm)"() -> (w514:dbl)
              n187 = local read "Target Z (µm)"() -> (w515:dbl)
              n188 = Index Array(array=w504, index=0) -> (element=w502:dbl)
              n189 = local write "Stage Position (µm)"(w502) -> ()
              n190 = Subtract(x=w502, y=w510) -> (x-y=w509:dbl)
              n191 = call "4Pi Focus Lock - Values Organize Plot Data.vi"("Target 01"=w515, "Value Limit"=w512, "Current 01"=w514, "Stage Position"=w509) -> ("output cluster"=→"Z Target and Fit Value (µm)":T1)  [unwired: 11 in]
            }
            frame "Abort" {
              n192 = Get Notifier Status(notifier=w521) -> (notifier out=w526:refnum<notifier>, current notification=w525:T3)  [unwired: 1 in, 3 out]
              n193 = call "Camera Messenger.vi"("Notifier Name"=w520, "General Camera Actions"=Generic_Camera_Actions."Abort") -> ()  [unwired: 8 in, 6 out]
              n194 = Bundle By Name(cluster=w525, "Running?"=FALSE, "Actions"=4Pi_Focus_Lock_-_Actions."Exit Loop") -> (w523:T3)
              n195 = Send Notification(notification=w523, notifier=w526) -> (notifier out=w517:refnum<notifier>)  [unwired: 1 in, 1 out]
            }
            frame "Exit Loop" {
            }
            frame "Quit" {
              n196 = Get Notifier Status(notifier=w532) -> (current notification=w539:T3)  [unwired: 1 in, 4 out]
              n197 = Unbundle By Name(w539) -> ("Ref Stack (SGL)"=w538:T4[], "Cur Image (SGL)"=w537:T4, "Tmp Image FFT (CSG)"=w536:T4, "Cur Image FFT (CSG)"=w535:T4, "CC Image (SGL)"=w534:T4, "Ref FFT Stack (CSG)"=w531:T4[], "Tmp Image1 FFT (CSG)"=w530:T4)
              n198 = Build Array (concatenate)(w538, w537, w536, w535, w534, w531, w530) -> (w533:T4[])
              n199 = for {
                tunnel: w533 -> [w542] mode=indexing
                n200 = call "IMAQ Dispose"("Image"=w542) -> ()  [unwired: 5 in, 1 out]
              }
            }
          }
          n201 = Get Notifier Status(notifier=w203) -> (current notification=w211:T3)  [unwired: 1 in, 4 out]
          n202 = Unbundle By Name(w211) -> ("Actions"=w210:T2)
          n203 = Equal?(x=w208, y=w210) -> (x = y?=w209:bool)
          n204 = Select(t=w208, s=w209, f=w207) -> (s? t:f=w206:T2)
        }
      }
      n205 = while {
        tunnel: w75 -> [w91]
        tunnel: w74 -> [w90]
        stop <- w89 stop-if-true
        n206 = event shown="[4] \"Start Lock\": Value Change" {
          selector: _ -> [_ _ _ _ _ _]
          dyn-events: _ -> [_ _ _ _ _ _]
          timeout: -1 -> [_ _ _ _ _ _]
          tunnel: w91 -> [_ w94 _ _ _ _]
          tunnel: w90 -> [_ _ w104 w141 w164 w168]
          tunnel: [w92 w93 w95 w137 w158 w166] -> w89
          tunnel: FALSE ("NewVal") -> [w92 w93 w95 w137 w158 _]
          event Timeout {
            n207 = event-data() -> ()  [unwired: 1 in, 3 out]
          }
          event "Set Camera ROI": Value Change {
            n208 = event-data() -> ()  [unwired: 1 in, 2 out]
            n209 = call "4Pi Focus Lock - Setup Camera.vi"("Camera Notifier Name"=w94) -> ()  [unwired: 14 in, 1 out]
          }
          event "P (Proportional)", "I (Integral)", "D (Derivative)", "Sample Z Step Size (µm)", "Z Move Limit (µm)", "Z Drift Threshold (µm)": Value Change {
            n210 = event-data() -> ("NewVal"=w99:dbl, "CtlRef"=w101:refnum<vi>)  [unwired: 1 in]
            n211 = Get Notifier Status(notifier=w104) -> (notifier out=w103:refnum<notifier>, current notification=w102:T3)  [unwired: 1 in, 3 out]
            n212 = property class="DigNum (strict)"(reference=w101) -> ("Label.Text"=w100:string)  [unwired: 1 in, 2 out]
            n213 = case shown="\"Z Drift Threshold (µm)\"" w100 {
              tunnel: w102 -> [w105 w108 w114 w120 w126 w129 w132]
              tunnel: w99 -> [_ w109 w115 w121 w125 w128 w131]
              tunnel: [w105 w106 w112 w118 w124 w127 w130] -> w98
              frame Default {
              }
              frame "P (Proportional)" {
                n214 = Unbundle By Name(w108) -> ("PID Values"=w110:dbl[])
                n215 = Replace Array Subset(array=w110, new element=w109, index=0) -> (w107:dbl[])
                n216 = Bundle By Name(cluster=w108, "PID Values"=w107) -> (w106:T3)
              }
              frame "I (Integral)" {
                n217 = Unbundle By Name(w114) -> ("PID Values"=w116:dbl[])
                n218 = Replace Array Subset(array=w116, new element=w115, index=1) -> (w113:dbl[])
                n219 = Bundle By Name(cluster=w114, "PID Values"=w113) -> (w112:T3)
              }
              frame "D (Derivative)" {
                n220 = Unbundle By Name(w120) -> ("PID Values"=w122:dbl[])
                n221 = Replace Array Subset(array=w122, new element=w121, index=2) -> (w119:dbl[])
                n222 = Bundle By Name(cluster=w120, "PID Values"=w119) -> (w118:T3)
              }
              frame "Sample Z Step Size (µm)" {
                n223 = Bundle By Name(cluster=w126, "Z Step Size (µm)"=w125) -> (w124:T3)
              }
              frame "Z Move Limit (µm)" {
                n224 = Bundle By Name(cluster=w129, "Z Stage Move Limit (µm)"=w128) -> (w127:T3)
              }
              frame "Z Drift Threshold (µm)" {
                n225 = Bundle By Name(cluster=w132, "Z Drift Threshold"=w131) -> (w130:T3)
              }
            }
            n226 = Bundle By Name(cluster=w98, "Actions"=4Pi_Focus_Lock_-_Actions."Idle") -> (w96:T3)
            n227 = Send Notification(notification=w96, notifier=w103) -> ()  [unwired: 1 in, 2 out]
          }
          event "Sample Z Step No.": Value Change {
            n228 = event-data() -> ("NewVal"=w135:u32)  [unwired: 1 in]
            n229 = Get Notifier Status(notifier=w141) -> (notifier out=w139:refnum<notifier>, current notification=w140:T3)  [unwired: 1 in, 3 out]
            n230 = for {
              N: w135 -> [_]
              tunnel: [w153] -> w134 mode=indexing
              tunnel: [w142] -> w133 mode=indexing
              i -> [w152]
              w143 = T5 3 items=["Grayscale (U8)", "Grayscale (I16)", "Grayscale (SGL)", "Complex (CSG)", "RGB (U32)", "HSL (U32)", "RGB (U64)", "Grayscale (U16)"] ("Image Type")
              w148 = T5 2 items=["Grayscale (U8)", "Grayscale (I16)", "Grayscale (SGL)", "Complex (CSG)", "RGB (U32)", "HSL (U32)", "RGB (U64)", "Grayscale (U16)"] ("Image Type")
              w144 = 10 ("Border Size")
              n231 = Number To Decimal String(number=w152, width (-)=i16 1) -> (decimal integer string=w150:string)
              n232 = Concatenate Strings("Ref Stack " ("string"), w150) -> (w146:string)
              n233 = call "IMAQ Create"("Border Size"=w144, "Image Name"=w146, "Image Type"=w148) -> ("New Image"=w153:T4)  [unwired: 2 in, 1 out]
              n234 = Concatenate Strings("FFT" ("string"), w146) -> (w145:string)
              n235 = call "IMAQ Create"("Border Size"=w144, "Image Name"=w145, "Image Type"=w143) -> ("New Image"=w142:T4)  [unwired: 2 in, 1 out]
            }
            n236 = Bundle By Name(cluster=w140, "Actions"=4Pi_Focus_Lock_-_Actions."Idle", "Z Step No."=w135, "Ref Stack (SGL)"=w134, "Ref FFT Stack (CSG)"=w133) -> (w138:T3)
            n237 = Send Notification(notification=w138, notifier=w139) -> ()  [unwired: 1 in, 2 out]
          }
          event "Start Lock": Value Change {
            n238 = event-data() -> ("NewVal"=w156:bool)  [unwired: 1 in]
            n239 = Select(t=4Pi_Focus_Lock_-_Actions."Start Lock", s=w156, f=4Pi_Focus_Lock_-_Actions."Abort" ("t")) -> (s? t:f=w161:T2)
            n240 = Select(t=TRUE ("Running?"), s=w156, f=FALSE) -> (s? t:f=w154:bool)
            n241 = Get Notifier Status(notifier=w164) -> (notifier out=w165:refnum<notifier>, current notification=w163:T3)  [unwired: 1 in, 3 out]
            n242 = Bundle By Name(cluster=w163, "Actions"=w161, "Running?"=w154) -> (w162:T3)
            n243 = Send Notification(notification=w162, notifier=w165) -> ()  [unwired: 1 in, 2 out]
          }
          event "Quit": Value Change {
            # "Turn off the Focus lock before quiting."
            n244 = event-data() -> ("NewVal"=w166:bool)  [unwired: 1 in]
            n245 = Get Notifier Status(notifier=w168) -> (notifier out=w171:refnum<notifier>, current notification=w169:T3)  [unwired: 1 in, 3 out]
            n246 = Unbundle By Name(w169) -> ("Running?"=w172:bool)
            n247 = case shown="False" w172 {
              tunnel: w171 -> [w176 w181]
              tunnel: [w176 w178] -> w170
              tunnel: w169 -> [_ w182]
              frame False {
              }
              frame True {
                n248 = Bundle By Name(cluster=w182, "Actions"=4Pi_Focus_Lock_-_Actions."Abort") -> (w180:T3)
                n249 = Send Notification(notification=w180, notifier=w181) -> (notifier out=w179:refnum<notifier>)  [unwired: 1 in, 1 out]
                n250 = while {
                  tunnel: w179 -> [w192]
                  tunnel: [w187] -> w178
                  i -> [w186]
                  stop <- w188 stop-if-true
                  n251 = Get Notifier Status(notifier=w192) -> (notifier out=w187:refnum<notifier>, # waiting=w191:i32)  [unwired: 1 in, 3 out]
                  n252 = Greater?(x=w186, y=1500) -> (0:w184:bool)
                  n253 = Less?(x=w191, y=1) -> (x < y?=w189:bool)
                  n254 = Or(x=w189, y=w184) -> (x .or. y?=w188:bool)
                  n255 = Wait (ms)(milliseconds to wait=u32 1) -> ()  [unwired: 1 out]
                }
              }
            }
            n256 = Get Notifier Status(notifier=w170) -> (notifier out=w174:refnum<notifier>, current notification=w175:T3)  [unwired: 1 in, 3 out]
            n257 = Bundle By Name(cluster=w175, "Actions"=4Pi_Focus_Lock_-_Actions."Quit") -> (w173:T3)
            n258 = Send Notification(notification=w173, notifier=w174) -> ()  [unwired: 1 in, 2 out]
          }
        }
      }
      n259 = Release Notifier(notifier=w72, force destroy? (F)=TRUE) -> ()  [unwired: 1 in, 3 out]
    }
    frame Error {
    }
  }
